vi "Target Align Errors.vi"(8 "Running Error Array":dbl[](array[numeric]), 11 "Running Phase Array":dbl[](array[numeric])) -> (3 "Error Table":dbl[](array[numeric]), 5 "Phase Table":dbl[](array[numeric]))   [LabVIEW 2018, in "COBRA Iterative Learning Control Library.lvlib"]
uses:
  COBRA Iterative Learning Control Library.lvlib
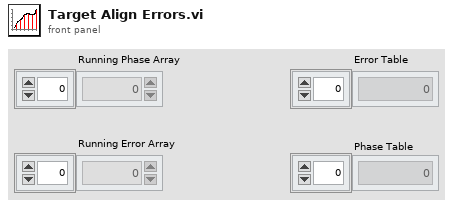
[diagram p1: front panel]
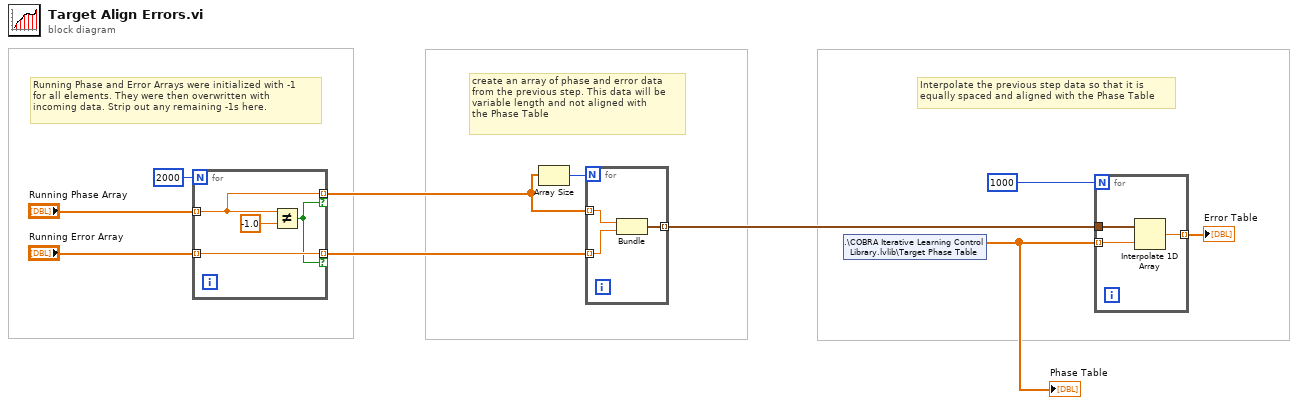
[diagram p0: block diagram]
diagram:
  # "Running Phase and Error Arrays were initialized with -1\nfor all elements. They were then overwritten with \nincoming data. Strip out any remaining -1s here."
  # "create an array of phase and error data\nfrom the previous step. This data will be \nvariable length and not aligned with\nthe Phase Table"
  # "Interpolate the previous step data so that it is\nequally spaced and aligned with the Phase Table"
  n1 = for {
    N: 2000 ("dimension size") -> [_]
    tunnel: "Running Phase Array" -> [w13] mode=indexing
    tunnel: "Running Error Array" -> [w12] mode=indexing
    tunnel: [w13] -> w8 mode=indexing if=w11
    tunnel: [w12] -> w6 mode=indexing if=w11
    n2 = Not Equal?(x=w13, y=-1.0) -> (x != y?=w11:bool)
  }
  n3 = Array Size(array=w8) -> (size(s)=w9:i32)
  n4 = for {
    N: w9 -> [_]
    tunnel: w8 -> [w17] mode=indexing
    tunnel: w6 -> [w16] mode=indexing
    tunnel: [w15] -> w7 mode=indexing
    n5 = Bundle("Numeric"=w17, "Numeric"=w16) -> (w15:cluster{"Numeric":dbl, "Numeric":dbl})  [unwired: 1 in]
  }
  n6 = shared-variable ".\\COBRA Iterative Learning Control Library.lvlib\\Target Phase Table"() -> (w5:dbl[])  [unwired: 1 in, 1 out]
  "Phase Table" <- w5
  n7 = for {
    N: 1000 -> [_]
    tunnel: w7 -> [w20]
    tunnel: w5 -> [w19] mode=indexing
    tunnel: [w18] -> w2 mode=indexing
    n8 = Interpolate 1D Array(1:w19, 2:w20) -> (0:w18:dbl)
  }
  "Error Table" <- w2
